vi "Configure test.vi"(6 "Assert VI Path":path, 7 "Existing Queue Elements":string, 8 "error in (no error)":errorcluster, 11 "Basic Test in":refnum<class "Test.lvclass">) -> (0 "error out":errorcluster, 3 "Test out":refnum<class "Test.lvclass">)   [LabVIEW 2018, in "Test.lvclass"]
uses:
  Test.lvclass
  f8dd1123-d8c2-47ee-b12c-874bd9b16366.vi
  292fa6e5-d529-4071-a2ec-9b26b6470a40.vi
  f8dd1123-d8c2-47ee-b12c-874bd9b16366.vi/76e2962b-4f71-41de-a834-6239a85fb408.vi
  f8dd1123-d8c2-47ee-b12c-874bd9b16366.vi/c5d19641-b18f-47fe-8e22-00db768ef2c6.vi
  <vilib>/JDP Science/JSONtext/String Subset.vi
  Test Class String IDs.vi
  <vilib>/JDP Science/JSONtext/Parsing/Parse Full Path or Item Name.vi
  <vilib>/JDP Science/JSONtext/Offset/Find Item Locations by Path.vi
  <vilib>/JDP Science/JSONtext/JSON text to Variant.vi
  <vilib>/JDP Science/JSONtext/Variant to JSON Text.vi
  <vilib>/JDP Science/JSONtext/Set Item.vi
  <vilib>/JDP Science/JSONtext/JSONtext.lvlib
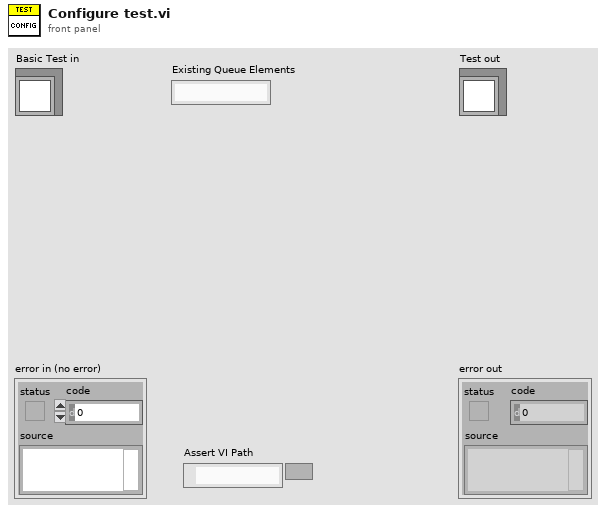
[diagram p1: front panel]
types:
  T1 = cluster{"Comparison Value 1":string, "Comparison Value 2":string, "Invert Result":string, "Assert VI Name":string, "Data Type":string, "Builder User Name":string, "Build Timestamp":string, "Failure Action":string, "Comment":string, "Assert Name":string, "Description":string, "Evaluation String":string}
  T2 = cluster{"Additional Data":string, "Comparison Value":string, "Invert?":string, "Assert Name":string, "Comment":string, "Default Failure Action":string, "Assert Build Timestamp":string, "Assert Builder User Name":string, "Data Type":string, "Assert VI Name":string, "Evaluation String":string}
  T3 = typedef "Icon Colours.ctl" = string
  T4 = typedef "NI_Data Type.lvlib/Data Type.ctl" = enum8{"Invalid Type", "Void", "I8", "I16", "I32", "I64", "U8", "U16", "U32", "U64", "Single Float", "Double Float", "Extended Float", "Single Complex", "Double Complex", "Extended Complex", "Enum U8", "Enum U16", "Enum U32", "Enum U64", "Single Float With Unit", "Double Float With Unit", "Extended Float With Unit", "Single Complex with Unit", "Double Complex with Unit", "Extended Complex with Unit", "Boolean", "String", "Path", "Picture", "Tag", "Array", "Cluster", "Variant", "LV Variant", "Waveform", "Timestamp", "Digital Waveform", "Digital Data", "ExpressData", "Refnum", "External Data", "VI", "Poly VI", "LabVIEW Class Instance", "Fixed Point"}
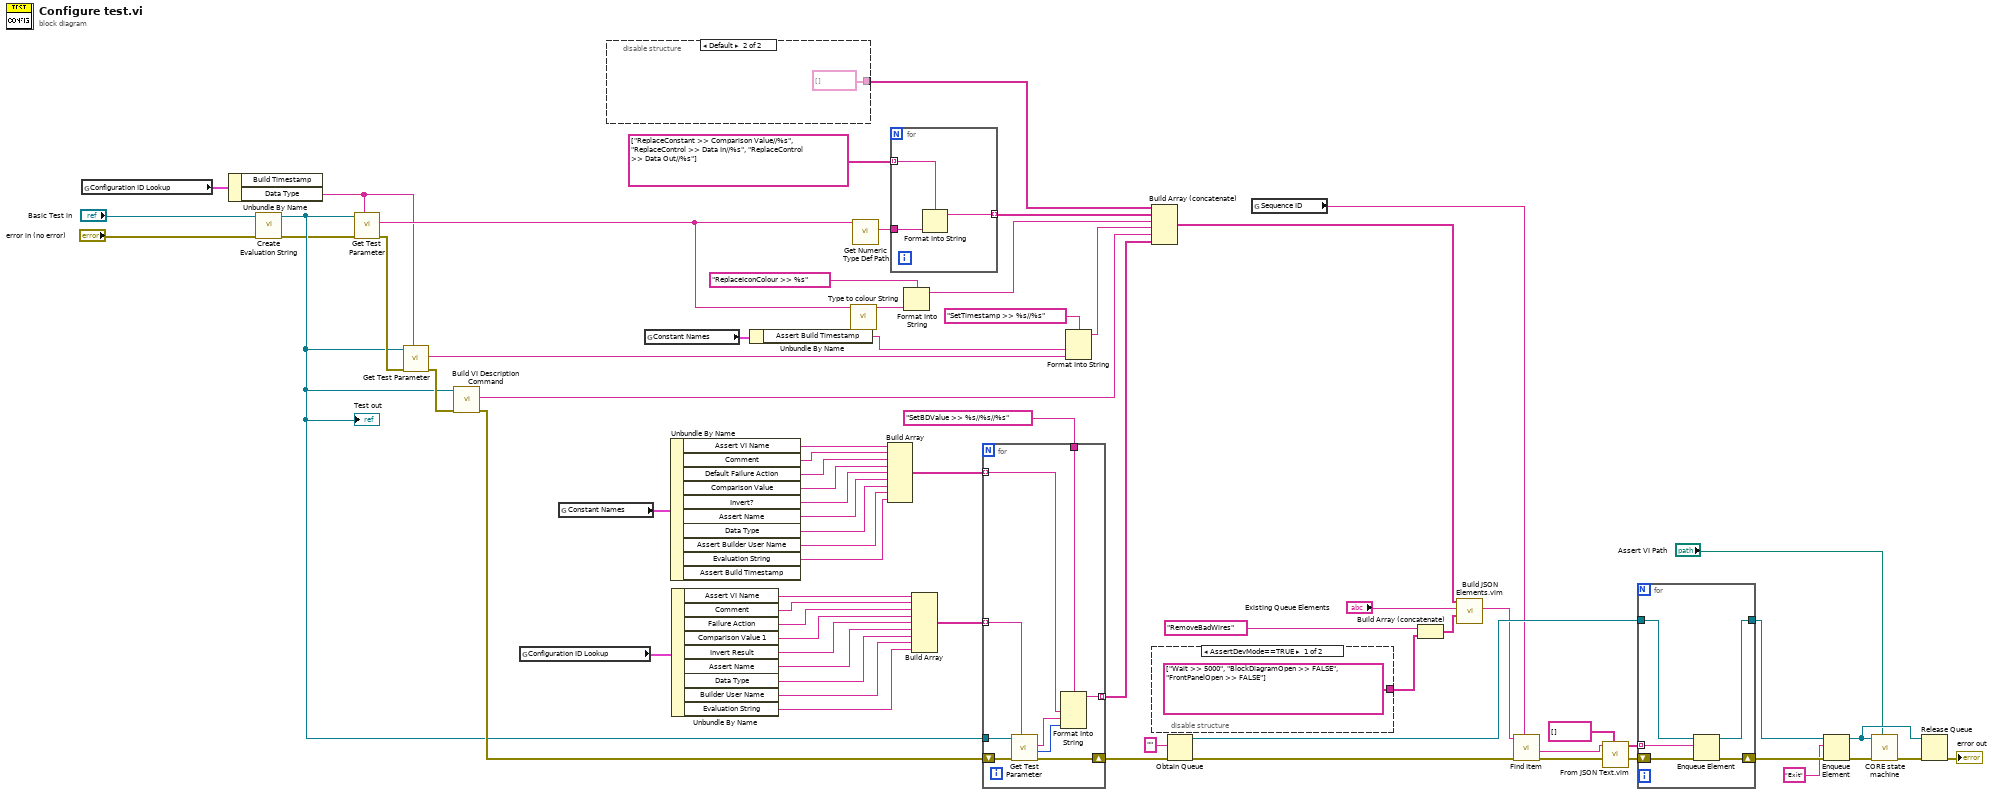
[diagram p0: block diagram]
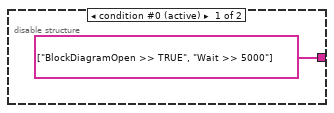
[diagram p3: hidden frame]
diagram:
  n1 = global read "Test Class String IDs.vi" "Configuration ID Lookup"() -> (w10:T1)
  n2 = Unbundle By Name(w10) -> ("Data Type"=w2:string)  [unwired: 1 out]
  n3 = call-dynamic "Create Evaluation String.vi"("error in (no error)"="error in (no error)", "Test in"="Basic Test in") -> ("error out"=w3:errorcluster, "Test out"=w11:refnum<class "Test.lvclass">)  [unwired: 8 in]
  "Test out" <- w11
  n4 = call "Get Test Parameter.vi"("Data Value ID"=w2, "error in (no error)"=w3, "Test in"=w11) -> ("error out"=w70:errorcluster, "Test Parameter"=w9:string)  [unwired: 6 in, 1 out]
  n5 = call "Get Test Parameter.vi"("Data Value ID"=w2, "error in (no error)"=w70, "Test in"=w11) -> ("error out"=w69:errorcluster, "Test Parameter"=w24:string)  [unwired: 6 in, 1 out]
  n6 = call "Build VI Description Command.vi"("error in (no error)"=w69, "Test in"=w11) -> ("error out"=w71:errorcluster, "VI Description Command"=w6:string)  [unwired: 8 in]
  n7 = global read "Test Class String IDs.vi" "Configuration ID Lookup"() -> (w42:T1)
  n8 = global read "Test Class String IDs.vi" "Constant Names"() -> (w41:T2)
  n9 = disable-structure shown="Default" {
    disable-tunnel: [string[] ["BlockDiagramOpen >> TRUE", "Wait >> 5000"] string[] []] -> w46
    frame condition #0 (active) {
    }
    frame condition #1 {
    }
  }
  n10 = global read "Test Class String IDs.vi" "Constant Names"() -> (w5:T2)
  n11 = Unbundle By Name(w41) -> ("Assert VI Name"=w39:string, "Comment"=w38:string, "Default Failure Action"=w37:string, "Comparison Value"=w36:string, "Invert?"=w35:string, "Assert Name"=w34:string, "Data Type"=w33:string, "Assert Builder User Name"=w32:string, "Evaluation String"=w19:string)  [unwired: 1 out]
  n12 = Unbundle By Name(w42) -> ("Assert VI Name"=w30:string, "Comment"=w29:string, "Failure Action"=w28:string, "Comparison Value 1"=w27:string, "Invert Result"=w26:string, "Assert Name"=w18:string, "Data Type"=w17:string, "Builder User Name"=w16:string, "Evaluation String"=w15:string)
  n13 = Unbundle By Name(w5) -> ("Assert Build Timestamp"=w4:string)
  n14 = call "Type to colour String.vi"("Type"=w9) -> ("Requested Colour"=w44:T3)  [unwired: 10 in]
  n15 = call "Get Numeric Type Def Path.vi"("Type"=w9) -> ("File Name"=w57:string)  [unwired: 9 in, 1 out]
  n16 = Build Array(w39, w38, w37, w36, w35, w34, w33, w32, w19) -> (w31:string[])
  n17 = for {
    tunnel: string[] ["ReplaceConstant >> Comparison Value//%s", "ReplaceControl >> Data In//%s", "ReplaceControl >> Data Out//%s"] -> [w76] mode=indexing
    tunnel: w57 -> [w75]
    tunnel: [w74] -> w48 mode=indexing
    n18 = Format Into String(format string=w76, w75) -> (resulting string=w74:string)  [unwired: 2 in, 1 out]
  }
  n19 = Format Into String(format string="ReplaceIconColour >> %s" ("String"), w44) -> (resulting string=w43:string)  [unwired: 2 in, 1 out]
  n20 = Build Array(w30, w29, w28, w27, w26, w18, w17, w16, w15) -> (w25:string[])
  n21 = for {
    tunnel: w11 -> [w83]
    tunnel: "SetBDValue >> %s//%s//%s" ("Append Element(s)") -> [w82]
    tunnel: [w81] -> w8 mode=indexing
    tunnel: w31 -> [w80] mode=indexing
    tunnel: w25 -> [w79] mode=indexing
    shift-right: [w77] -> w20
    shift-left: w71 -> [w78]
    n22 = call "Get Test Parameter.vi"("Data Value ID"=w79, "error in (no error)"=w78, "Test in"=w83) -> ("error out"=w77:errorcluster, "Data Type"=w84:T4, "Test Parameter"=w85:string)  [unwired: 6 in]
    n23 = Format Into String(format string=w82, w80, w85, w84) -> (resulting string=w81:string)  [unwired: 2 in, 1 out]
  }
  n24 = Format Into String(format string="SetTimestamp >> %s//%s" ("Append Element(s)"), w4, w24) -> (resulting string=w7:string)  [unwired: 2 in, 1 out]
  n25 = Build Array (concatenate)(w46, w48, w43, w7, w6, w8) -> (w47:string[])
  n26 = disable-structure shown="AssertDevMode==TRUE" {
    disable-tunnel: [string[] ["Wait >> 5000", "BlockDiagramOpen >> FALSE", "FrontPanelOpen >> FALSE"] _] -> w14
    frame condition #0 (active) {
    }
    frame condition #1 {
    }
  }
  n27 = Obtain Queue(element data type="", error in (no error)=w20) -> (queue out=w67:refnum<queue>, error out=w66:errorcluster)  [unwired: 3 in, 1 out]
  n28 = global read "Test Class String IDs.vi" "Sequence ID"() -> (w49:string)
  n29 = Build Array (concatenate)("RemoveBadWires" ("String"), w14) -> (w12:string[])
  n30 = call "Build JSON Elements.vim"("Append Element(s)"=w12, "JSON Elements in ({})"="Existing Queue Elements", "Prepend Element(s)"=w47) -> ("JSON Elements out"=w55:string)  [unwired: 8 in]
  n31 = call <vilib>:"Find Item.vi"("$Path or Item Name"=w49, "error in (no error)"=w66, "JSON"=w55) -> ("error out"=w52:errorcluster, "<JSON>"=w54:string)  [unwired: 5 in, 2 out]
  n32 = call "From JSON Text.vim"("Data Type and Default Value"=string[] [], "error in (no error)"=w52, "JSON"=w54) -> ("error out"=w50:errorcluster, "Data out"=w51:string[])  [unwired: 7 in]
  n33 = for {
    tunnel: w51 -> [w89] mode=indexing
    tunnel: w67 -> [w91]
    shift-right: [w87] -> w65
    shift-left: w50 -> [w90]
    tunnel: [w88] -> w63
    n34 = Enqueue Element(queue=w91, element=w89, error in (no error)=w90) -> (queue out=w88:refnum<queue>, error out=w87:errorcluster)  [unwired: 1 in, 1 out]
  }
  n35 = Enqueue Element(queue=w63, element="Exit", error in (no error)=w65) -> (queue out=w59:refnum<queue>, error out=w64:errorcluster)  [unwired: 1 in, 1 out]
  n36 = call "CORE state machine.vi"("Assert VI Path"="Assert VI Path", "error in (no error)"=w64, "State Machine Queue"=w59) -> ("error out"=w61:errorcluster)  [unwired: 8 in]
  n37 = Release Queue(queue=w59, error in (no error)=w61) -> (error out=→"error out":errorcluster)  [unwired: 1 in, 2 out]
